vi "Parse 18-1.vi"(11 "Input":string) -> (3 "Numbers":refnum<class "SnailNum.lvclass">[](array[class]))   [LabVIEW 2020]
uses:
  SnailNum/SnailNum.lvclass
panel:
  out "To String":string[](array[string])
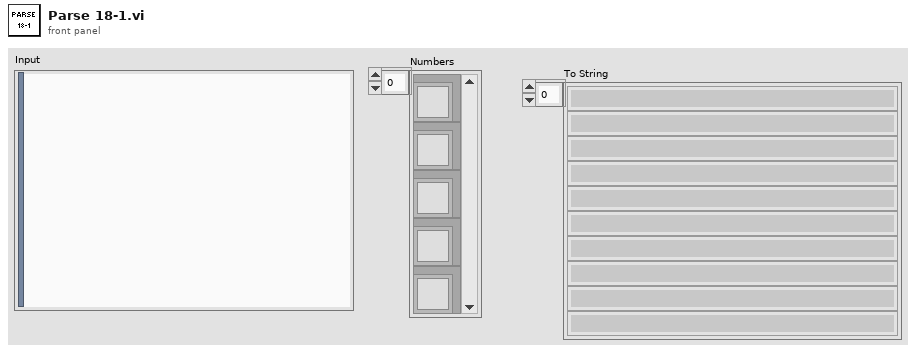
[diagram p1: front panel]
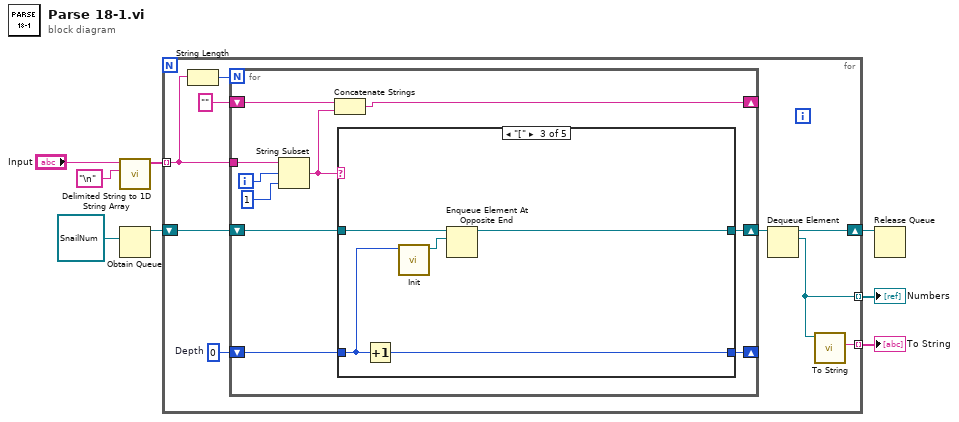
[diagram p0: block diagram]
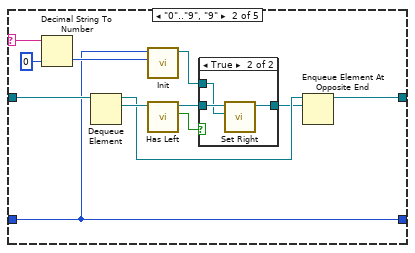
[diagram p3: hidden frame]
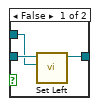
[diagram p4: hidden frame]
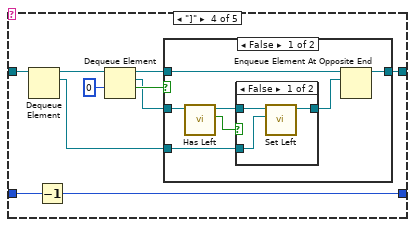
[diagram p5: hidden frame]
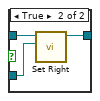
[diagram p6: hidden frame]
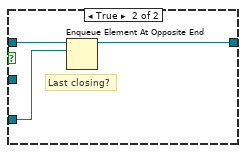
[diagram p7: hidden frame]
diagram:
  n1 = call <vilib>:"Delimited String to 1D String Array.vi"("delimiter"="\n", "delimited string"="Input") -> ("string array"=w8:string[])  [unwired: 9 in]
  n2 = Obtain Queue(element data type=refnum<class "SnailNum.lvclass"> refnum ("Current")) -> (queue out=w5:refnum<queue>)  [unwired: 4 in, 2 out]
  n3 = for {
    tunnel: w8 -> [w16] mode=indexing
    shift-right: [w11] -> w4
    shift-left: w5 -> [w15]
    tunnel: [w10] -> w3 mode=indexing
    tunnel: [w9] -> w1 mode=indexing
    w13 = 0  # Depth
    n4 = String Length(string=w16) -> (length=w17:i32)
    n5 = for {
      N: w17 -> [_]
      tunnel: w16 -> [w27]
      shift-right: [w23] -> w14
      shift-left: w15 -> [w24]
      shift-right: [w21] -> _
      shift-left: w13 -> [w22]
      shift-right: [w18] -> _
      shift-left: "" -> [w20]
      i -> [w26]
      n6 = String Subset(string=w27, offset (0)=w26, length (rest)=1 ("length (rest)")) -> (substring=w19:string)
      n7 = Concatenate Strings(w20, w19) -> (w18:string)
      n8 = case shown="\"[\"" w19 {
        selector: w19 -> [_ w37 _ _ _]
        tunnel: w24 -> [w29 w41 w52 w62 w80]
        tunnel: [w29 w33 w51 w57 w80] -> w23
        tunnel: w22 -> [w28 w30 w48 w54 w79]
        tunnel: [w28 w30 w50 w53 w79] -> w21
        frame Default {
        }
        frame "0".."9", "9" {
          n9 = Decimal String To Number(string=w37, default (0L)=i64 0) -> (number=w32:i64)  [unwired: 1 in, 1 out]
          n10 = Dequeue Element(queue=w41) -> (queue out=w35:refnum<queue>, element=w40:refnum<class "SnailNum.lvclass">)  [unwired: 2 in, 2 out]
          n11 = call "Init.vi"("Value"=w32, "Depth"=w30) -> ("SnailNum out"=w31:refnum<class "SnailNum.lvclass">)  [unwired: 8 in, 1 out]
          n12 = call "Has Left.vi"("SnailNum in"=w40) -> ("Has Left"=w39:bool, "SnailNum out"=w38:refnum<class "SnailNum.lvclass">)  [unwired: 8 in, 1 out]
          n13 = case shown="True" w39 {
            tunnel: w38 -> [w44 w47]
            tunnel: w31 -> [w43 w46]
            tunnel: [w42 w45] -> w34
            frame False {
              n14 = call "Set Left.vi"("Left"=w43, "SnailNum in"=w44) -> ("SnailNum out"=w42:refnum<class "SnailNum.lvclass">)  [unwired: 8 in, 1 out]
            }
            frame True {
              n15 = call "Set Right.vi"("Right"=w46, "SnailNum in"=w47) -> ("SnailNum out"=w45:refnum<class "SnailNum.lvclass">)  [unwired: 8 in, 1 out]
            }
          }
          n16 = Enqueue Element At Opposite End(queue=w35, element=w34) -> (queue out=w33:refnum<queue>)  [unwired: 2 in, 2 out]
        }
        frame "[" {
          n17 = Increment(x=w48) -> (x+1=w50:i32)
          n18 = call "Init.vi"("Depth"=w48) -> ("SnailNum out"=w49:refnum<class "SnailNum.lvclass">)  [unwired: 9 in, 1 out]
          n19 = Enqueue Element At Opposite End(queue=w52, element=w49) -> (queue out=w51:refnum<queue>)  [unwired: 2 in, 2 out]
        }
        frame "]" {
          n20 = Dequeue Element(queue=w62) -> (queue out=w61:refnum<queue>, element=w56:refnum<class "SnailNum.lvclass">)  [unwired: 2 in, 2 out]
          n21 = Decrement(x=w54) -> (x-1=w53:i32)
          n22 = Dequeue Element(queue=w61, timeout in ms (-1)=0) -> (queue out=w58:refnum<queue>, element=w55:refnum<class "SnailNum.lvclass">, timed out?=w59:bool)  [unwired: 1 in, 1 out]
          n23 = case shown="False" w59 {
            tunnel: w58 -> [w69 w78]
            tunnel: [w68 w76] -> w57
            tunnel: w56 -> [w64 w77]
            tunnel: w55 -> [w67 _]
            frame False {
              n24 = call "Has Left.vi"("SnailNum in"=w67) -> ("Has Left"=w66:bool, "SnailNum out"=w65:refnum<class "SnailNum.lvclass">)  [unwired: 8 in, 1 out]
              n25 = case shown="False" w66 {
                tunnel: w65 -> [w72 w75]
                tunnel: w64 -> [w70 w74]
                tunnel: [w71 w73] -> w63
                frame False {
                  n26 = call "Set Left.vi"("Left"=w70, "SnailNum in"=w72) -> ("SnailNum out"=w71:refnum<class "SnailNum.lvclass">)  [unwired: 8 in, 1 out]
                }
                frame True {
                  n27 = call "Set Right.vi"("Right"=w74, "SnailNum in"=w75) -> ("SnailNum out"=w73:refnum<class "SnailNum.lvclass">)  [unwired: 8 in, 1 out]
                }
              }
              n28 = Enqueue Element At Opposite End(queue=w69, element=w63) -> (queue out=w68:refnum<queue>)  [unwired: 2 in, 2 out]
            }
            frame True {
              # "Last closing?"
              n29 = Enqueue Element At Opposite End(queue=w78, element=w77) -> (queue out=w76:refnum<queue>)  [unwired: 2 in, 2 out]
            }
          }
        }
        frame "," {
        }
      }
    }
    n30 = Dequeue Element(queue=w14) -> (queue out=w11:refnum<queue>, element=w10:refnum<class "SnailNum.lvclass">)  [unwired: 2 in, 2 out]
    n31 = call "To String.vi"("SnailNum in"=w10) -> ("String"=w9:string)  [unwired: 8 in, 2 out]
  }
  "Numbers" <- w3
  "To String" <- w1
  n32 = Release Queue(queue=w4) -> ()  [unwired: 2 in, 3 out]
